vi "Init.vi"(11 "Input":string="Monkey 0:\n  Starting items: 93, 98\n  Operation: new = old * 17\n  Test: divisible by 19\n    If true: throw to monkey 5\n    If false: throw to monkey 3") -> (3 "Monkey":refnum<class "Monkey.lvclass">)   [LabVIEW 2022 SP3, in "AoC22.lvlib" / "Monkey.lvclass"]
uses:
  Monkey.lvclass
  Op.ctl
  Monkey.lvclass/Monkey.ctl
  <vilib>/Utility/error.llb/Trim Whitespace One-Sided.vi
  <vilib>/IlluminatedG/lv-stream/Stream.lvlib
  Worry Level.ctl
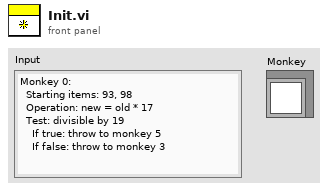
[diagram p1: front panel]
types:
  T1 = typedef "AoC22.lvlib/Monkey.lvclass/Op.ctl" = enum16{"+", "*"}
  T2 = typedef "AoC22.lvlib/Monkey.lvclass/Worry Level.ctl" = ext
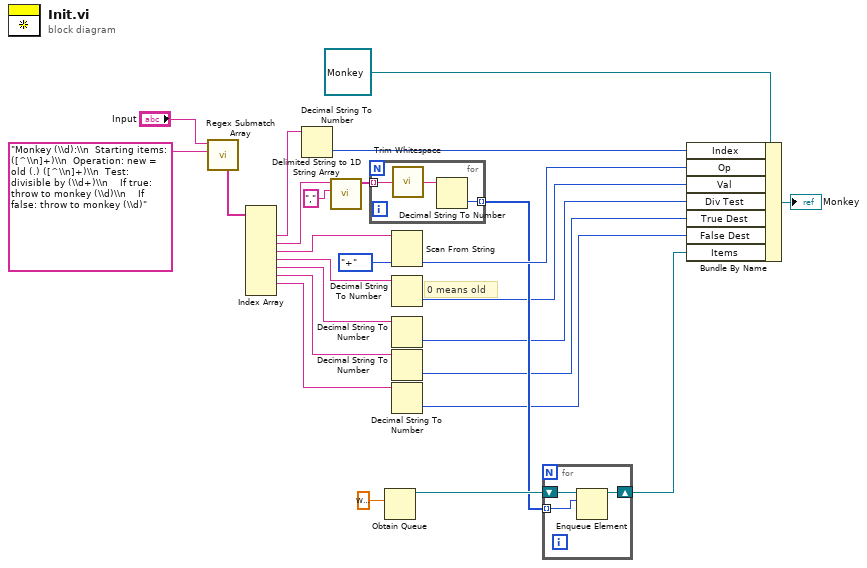
[diagram p0: block diagram]
diagram:
  # "0 means old"
  n1 = call <vilib>:"Regex Submatch Array.vi"("regular expression"="Monkey (\\d):\\n  Starting items: ([^\\n]+)\\n  Operation: new = old (.) ([^\\n]+)\\n  Test: divisible by (\\d+)\\n    If true: throw to monkey (\\d)\\n    If false: throw to monkey (\\d)", "string"="Input") -> ("matches"=w22:string[])  [unwired: 7 in, 2 out]
  n2 = Index Array(array=w22) -> (element #2=w21:string, element #3=w18:string, element #4=w14:string, element #5=w9:string, element #6=w7:string, element #7=w5:string, element #8=w2:string)  [unwired: 9 in, 2 out]
  n3 = Decimal String To Number(string=w21) -> (number=w19:i32)  [unwired: 2 in, 1 out]
  n4 = call <vilib>:"Delimited String to 1D String Array.vi"("delimiter"=",", "delimited string"=w18) -> ("string array"=w16:string[])  [unwired: 9 in]
  n5 = for {
    tunnel: w16 -> [w28] mode=indexing
    tunnel: [w26] -> w11 mode=indexing
    n6 = call <vilib>:"Trim Whitespace.vi"("string"=w28) -> ("trimmed string"=w27:string)  [unwired: 1 in]
    n7 = Decimal String To Number(string=w27) -> (number=w26:i32)  [unwired: 2 in, 1 out]
  }
  n8 = Obtain Queue(element data type=T2 0.0) -> (queue out=w12:refnum<queue>)  [unwired: 4 in, 2 out]
  n9 = Scan From String(input string=w14, default 1=Op."+" ("Operation.Op")) -> (output 1=w13:T1)  [unwired: 3 in, 3 out]
  n10 = Decimal String To Number(string=w9) -> (number=w8:i32)  [unwired: 2 in, 1 out]
  n11 = Decimal String To Number(string=w7) -> (number=w6:i32)  [unwired: 2 in, 1 out]
  n12 = Decimal String To Number(string=w5) -> (number=w4:i32)  [unwired: 2 in, 1 out]
  n13 = Decimal String To Number(string=w2) -> (number=w1:i32)  [unwired: 2 in, 1 out]
  n14 = for {
    shift-right: [w29] -> w10
    shift-left: w12 -> [w31]
    tunnel: w11 -> [w30] mode=indexing
    n15 = Enqueue Element(queue=w31, element=w30) -> (queue out=w29:refnum<queue>)  [unwired: 2 in, 2 out]
  }
  n16 = Bundle By Name(cluster=refnum<class "Monkey.lvclass"> refnum ("AoC22.lvlib:Monkey.lvclass"), "Index"=w19, "Op"=w13, "Val"=w8, "Div Test"=w6, "True Dest"=w4, "False Dest"=w1, "Items"=w10) -> (→"Monkey":refnum<class "Monkey.lvclass">)
